vi "Initialize.vi"(8 "error in (no error)":errorcluster, 9 "Requestor":string, 10 "Requestee":string, 11 "Compound Measurement in":refnum<class "Compound Measurement.lvclass">) -> (0 "error out":errorcluster, 3 "Compound Measurement out":refnum<class "Compound Measurement.lvclass">)   [LabVIEW 2015, in "Compound Measurement.lvclass"]
uses:
  Compound Measurement.lvclass
  Mag Lab Root/Mag Lab Root.lvclass/Mag Lab Root.ctl
  <vilib>/ActorFramework/Actor/Actor.lvclass/Actor.ctl
  <vilib>/ActorFramework/Message Enqueuer/Message Enqueuer.lvclass/Message Enqueuer.ctl
  Compound Measurement.lvclass/Compound Measurement.ctl
  Mag Lab Result/Mag Lab Result.lvclass
  Mag Lab Root Messages/Initialize Msg/Initialize Msg.lvclass/Initialize Msg.ctl
  <vilib>/ActorFramework/Message Enqueuer/Init from Existing Queue.vi
  <vilib>/ActorFramework/Message Enqueuer/Enqueue.vi
  <vilib>/ActorFramework/Message Priority Queue/Priority Enqueue.vi
  <vilib>/ActorFramework/Message Enqueuer/Message Enqueuer.lvclass
  Mag Lab Root Messages/Initialize Msg/Initialize Msg.lvclass
  <vilib>/ActorFramework/Actor/Actor.lvclass
  Mag Lab Root/Mag Lab Root.lvclass
  Mag Lab Error Handler/Mag Lab Error Handler.lvclass
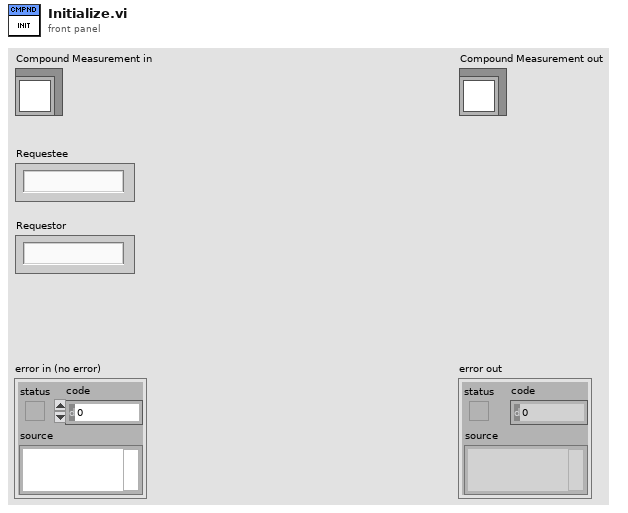
[diagram p1: front panel]
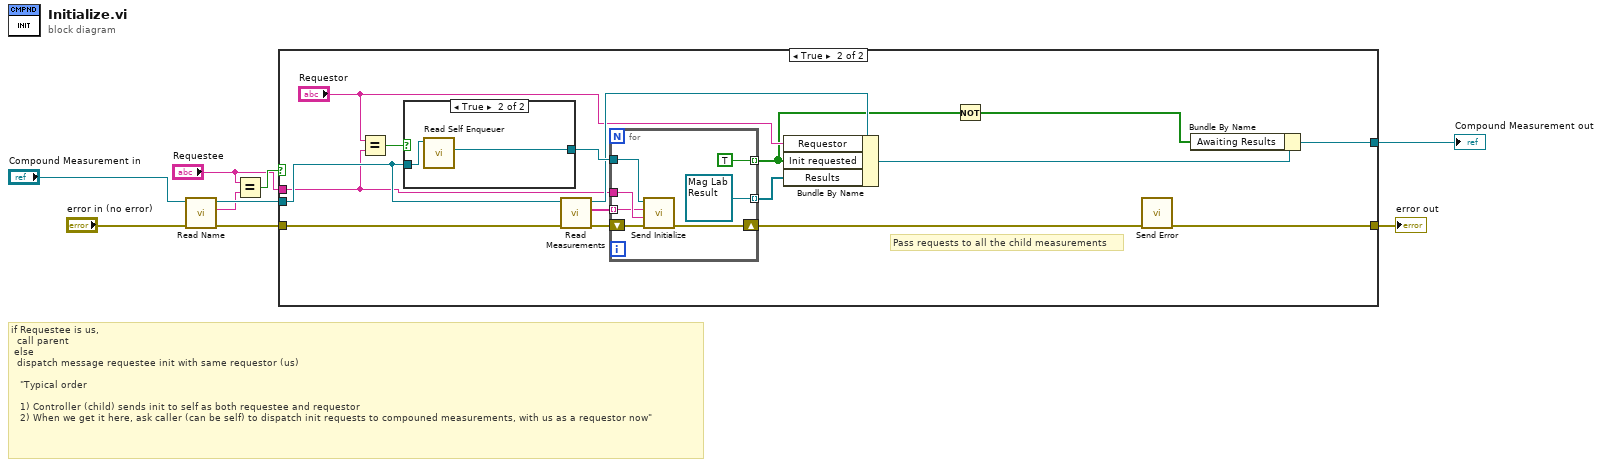
[diagram p0: block diagram]
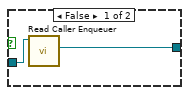
[diagram p3: hidden frame]
diagram:
  # "if Requestee is us, \n\t\tcall parent\n\telse\n\t\tdispatch message requestee init with same requestor (us)\n\n\t\t\t\"Typical order\n\n\t\t\t1) Controller (child) sends init to self as both requestee and requestor\n\t\t\t2) When we get it here, ask caller (can be self) to dispatch init requests to compouned measurements, with us as a requestor now\""
  n1 = call "Read Name.vi"("error in (no error)"="error in (no error)", "Mag Lab Root in"="Compound Measurement in") -> ("error out"=w6:errorcluster, "Name"=w2:string, "Mag Lab Root out"=w7:refnum<class "Compound Measurement.lvclass">)  [unwired: 7 in]
  n2 = Equal?(x="Requestee", y=w2) -> (x = y?=w4:bool)
  n3 = case shown="True" w4 {
    tunnel: "Requestee" -> [_ w20]
    tunnel: [w11 w16] -> w9
    tunnel: w6 -> [w10 w24]
    tunnel: w7 -> [w11 w23]
    tunnel: [w10 w18] -> w3
    frame False {
      # "Assumes we are the controller, bypass this than, avoid looping requests back"
    }
    frame True {
      # "Pass requests to all the child measurements"
      n4 = Equal?(x="Requestor", y=w20) -> (x = y?=w21:bool)
      n5 = case shown="True" w21 {
        tunnel: [w29 w31] -> w26
        tunnel: w23 -> [w28 w30]
        frame False {
          n6 = call <vilib>:"Read Caller Enqueuer.vi"("Actor"=w28) -> ("Caller Enqueuer"=w29:refnum<class "Message Enqueuer.lvclass">)  [unwired: 10 in]
        }
        frame True {
          n7 = call <vilib>:"Read Self Enqueuer.vi"("Actor"=w30) -> ("Self Enqueuer"=w31:refnum<class "Message Enqueuer.lvclass">)  [unwired: 10 in]
        }
      }
      n8 = call "Read Measurements.vi"("error in (no error)"=w24, "Compound Measurement in"=w23) -> ("error out"=w25:errorcluster, "Measurements"=w27:string[], "Compound Measurement out"=w22:refnum<class "Compound Measurement.lvclass">)  [unwired: 7 in]
      n9 = for {
        tunnel: w27 -> [w36] mode=indexing
        tunnel: w26 -> [w38]
        tunnel: w20 -> [w37]
        shift-right: [w34] -> w13
        shift-left: w25 -> [w35]
        tunnel: [TRUE] -> w15 mode=indexing
        tunnel: [refnum<class "Mag Lab Result.lvclass"> refnum ("Mag Lab Result.lvclass")] -> w17 mode=indexing
        n10 = call "Send Initialize.vi"("error in (no error)"=w35, "Requestor"=w37, "Requestee"=w36, "Message Enqueuer"=w38) -> ("error out"=w34:errorcluster)  [unwired: 6 in, 1 out]
      }
      n11 = Bundle By Name(cluster=w22, "Requestor"="Requestor", "Init requested"=w15, "Results"=w17) -> (w14:refnum<class "Compound Measurement.lvclass">)
      n12 = Not(x=w15) -> (.not. x?=w12:bool[])
      n13 = call "Send Error.vi"("error in (no error)"=w13) -> ("error out"=w18:errorcluster)  [unwired: 9 in, 1 out]
      n14 = Bundle By Name(cluster=w14, "Awaiting Results"=w12) -> (w16:refnum<class "Compound Measurement.lvclass">)
    }
  }
  "Compound Measurement out" <- w9
  "error out" <- w3
